vi "Setting Voltage & load.vi"(5 "N_Voltage":i32=3, 6 "Min_Power [W]":dbl=50.0 format="%0.2f", 7 "Max_Voltage [V]":dbl=5.0 format="%0.2f", 8 "Max_Power [W]":dbl=100.0 format="%0.2f", 9 "N_Power":i32=3, 10 "Min_Voltage [V]":dbl=2.5 format="%0.2f") -> (1 "Powers":dbl[](array[numeric]), 2 "Voltages":dbl[](array[numeric]))   [LabVIEW 2018]
uses:
  <vilib>/Analysis/NI_AALBase.lvlib
  <vilib>/Analysis/1siggen.llb/Ramp Pattern by Samples.vi
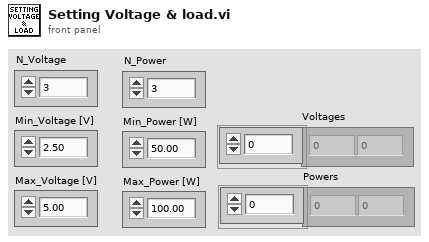
[diagram p1: front panel]
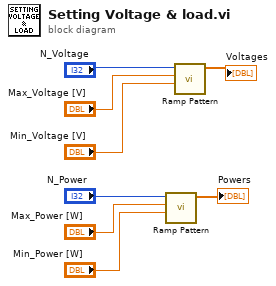
[diagram p0: block diagram]
diagram:
  n1 = call-poly <vilib>:"Ramp Pattern.vi"("start"="Min_Power [W]", "end"="Max_Power [W]", "samples"="N_Power") -> ("Ramp Pattern"=→"Powers":dbl[])  [unwired: 7 in, 1 out]
  n2 = call-poly <vilib>:"Ramp Pattern.vi"("start"="Min_Voltage [V]", "end"="Max_Voltage [V]", "samples"="N_Voltage") -> ("Ramp Pattern"=→"Voltages":dbl[])  [unwired: 7 in, 1 out]
